vi "Variant_GetArrayElementTypeDescriptor.vi"(7 "Name Element if empty string (F)":bool, 11 "Array":variant) -> (2 "Element Name":string, 3 "Element Descriptor":i16[](array[numeric]) format="%04x")   [LabVIEW 2013]
uses:
  TypeDescriptor/TypeDescriptor_GetPString.vi
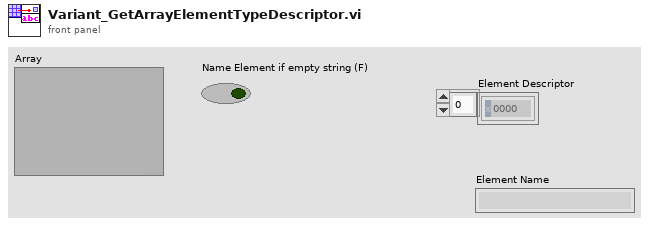
[diagram p1: front panel]
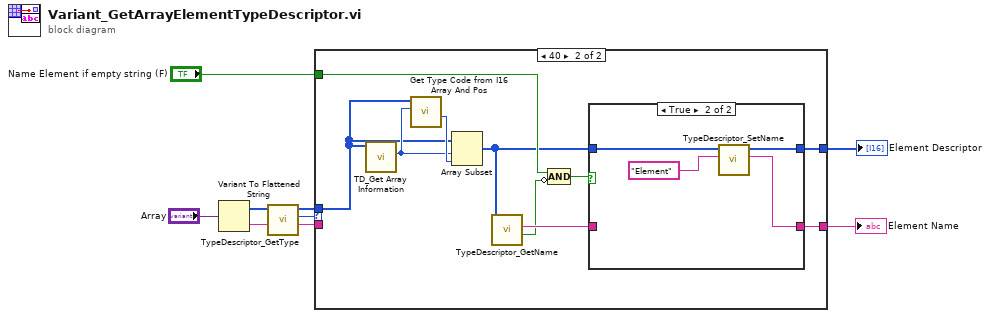
[diagram p0: block diagram]
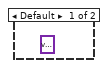
[diagram p2: hidden frame]
diagram:
  n1 = Variant To Flattened String(Variant="Array") -> (data string=w6:string, 1:w1:i16[])
  n2 = call "TypeDescriptor_GetType.vi"("type descriptor"=w1) -> ("Type"=w4:u8, "type descriptor dup"=w5:i16[])  [unwired: 9 in]
  n3 = case shown="40" w4 {
    tunnel: [_ w14] -> w7
    tunnel: w6 -> [_ _]
    tunnel: w5 -> [_ w16]
    tunnel: [_ w9] -> w3
    tunnel: "Name Element if empty string (F)" -> [_ w13]
    frame Default {
      (unwired) variant ("Default Element")
    }
    frame 64 {
      n4 = call <vilib>:"TD_Get Array Information.vi"("Type descriptor"=w16) -> ("Contained TD Offset"=w17:i32)  [unwired: 8 in, 2 out]
      n5 = call <vilib>:"Get Type Code from I16 Array And Pos.vi"("Pos in Type Descriptor (0)"=w17, "Type descriptor"=w16) -> ("Size (Words)"=w18:i32)  [unwired: 7 in, 2 out]
      n6 = Array Subset(array=w16, index=w17, length=w18) -> (w10:i16[])
      n7 = call "TypeDescriptor_GetName.vi"("type descriptor"=w10) -> ("found"=w12:bool, "name"=w15:string)  [unwired: 8 in, 1 out]
      n8 = Compound Arithmetic op=AND(w13, invert w12) -> (w11:bool)
      n9 = case shown="True" w11 {
        tunnel: w15 -> [w19 _]
        tunnel: [w19 w21] -> w14
        tunnel: w10 -> [w20 w23]
        tunnel: [w20 w24] -> w9
        frame False {
        }
        frame True {
          n10 = call "TypeDescriptor_SetName.vi"("name"="Element" ("format string"), "type descriptor"=w23) -> ("name out"=w21:string, "type descriptor dup"=w24:i16[])  [unwired: 7 in, 1 out]
        }
      }
    }
  }
  "Element Descriptor" <- w3
  "Element Name" <- w7
